vi "createLibrary.vi"(8 "error in (no error)":errorcluster, 10 "directoryPath":path, 11 "Module in":refnum<class "Module.lvclass">) -> (0 "error out":errorcluster, 3 "Module out":refnum<class "Module.lvclass">)   [LabVIEW 2013, in "Module.lvclass"]
uses:
  Module.lvclass
  Module.lvclass/Module.ctl
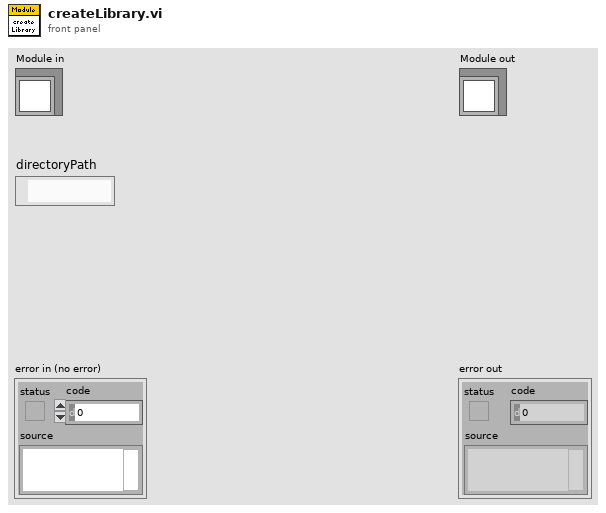
[diagram p1: front panel]
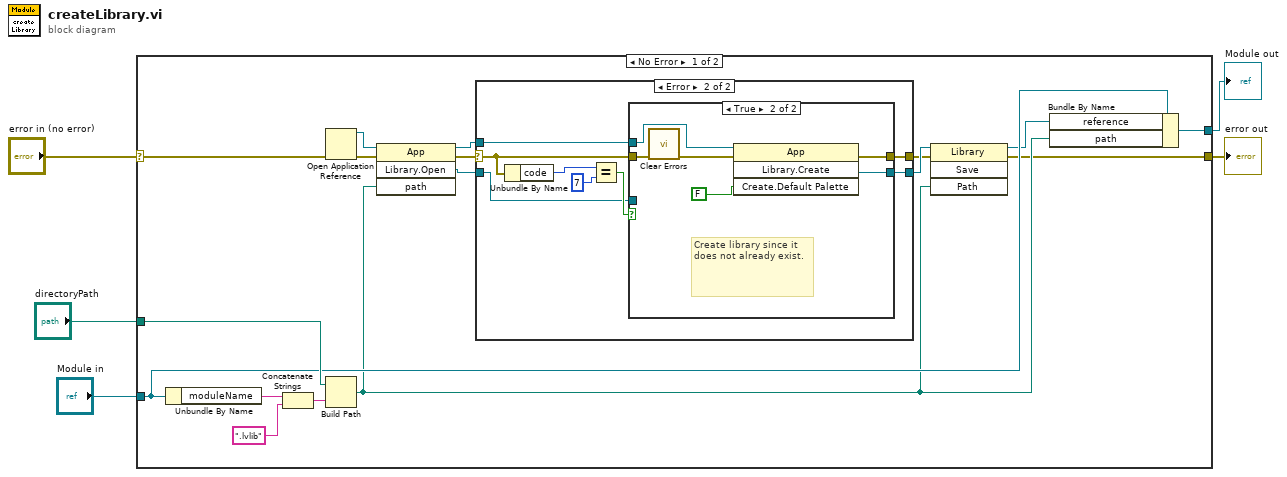
[diagram p0: block diagram]
diagram:
  n1 = case shown="No Error" "error in (no error)" {
    selector: "error in (no error)" -> [w12 w42]
    tunnel: [w6 w42] -> w4
    tunnel: [w17 w41] -> w2
    tunnel: "Module in" -> [w18 w41]
    tunnel: "directoryPath" -> [w19 _]
    frame No Error {
      n2 = Unbundle By Name(w18) -> ("moduleName"=w20:string)
      n3 = Concatenate Strings(w20, ".lvlib" ("string")) -> (w22:string)
      n4 = Open Application Reference(8:w12) -> (0:w13:errorcluster, 3:w15:refnum<vi>)  [unwired: 3 in]
      n5 = Build Path(base path=w19, name or relative path=w22) -> (appended path=w14:path)
      n6 = invoke class="App" method="Library.Open"(reference=w15, error in=w13, "path"=w14) -> (reference out=w10:refnum<vi>, error out=w11:errorcluster, "Open Library"=w7:refnum<vi>)  [unwired: 1 in, 1 out]
      n7 = case shown="Error" w11 {
        selector: w11 -> [w24 w29]
        tunnel: [w24 w28] -> w8
        tunnel: w10 -> [_ w27]
        tunnel: [w23 w26] -> w9
        tunnel: w7 -> [w23 w25]
        frame No Error {
        }
        frame Error {
          n8 = Unbundle By Name(w29) -> ("code"=w32:i32)
          n9 = Equal?(x=w32, y=7) -> (x = y?=w30:bool)
          n10 = case shown="True" w30 {
            tunnel: w29 -> [w34 w40]
            tunnel: [w34 w36] -> w28
            tunnel: w27 -> [_ w37]
            tunnel: [w33 w35] -> w26
            tunnel: w25 -> [w33 _]
            frame False {
            }
            frame True {
              # "Create library since it does not already exist."
              n11 = call <vilib>:"Clear Errors.vi"("error in (no error)"=w40) -> ("error out"=w38:errorcluster)  [unwired: 6 in]
              n12 = invoke class="App" method="Library.Create"(reference=w37, error in=w38, "Create.Default Palette"=FALSE ("Create:Default Palette")) -> (error out=w36:errorcluster, "Create Library"=w35:refnum<vi>)  [unwired: 1 in, 2 out]
            }
          }
        }
      }
      n13 = invoke class="Library" method="Save"(reference=w9, error in=w8, "Path"=w14) -> (reference out=w16:refnum<vi>, error out=w6:errorcluster)  [unwired: 1 in, 2 out]
      n14 = Bundle By Name(cluster=w18, "reference"=w16, "path"=w14) -> (w17:refnum<class "Module.lvclass">)
    }
    frame Error {
    }
  }
  "error out" <- w4
  "Module out" <- w2
